vi "PH_PILS.enable extExp.vi"(0 "i ref in":refnum<vi>, 2 "Experiment.Experiment":T1(ring), 5 "error in":errorcluster) -> (14 "i ref out":refnum<vi>, 19 "error out":errorcluster)   [LabVIEW 2014, in "PH_PILS.lvlib"]
uses:
  PH_PILS.lvlib
  PH_Common/PH_Common.lvlib
  PH_SystemInformation/PH_SystemInformation.lvlib
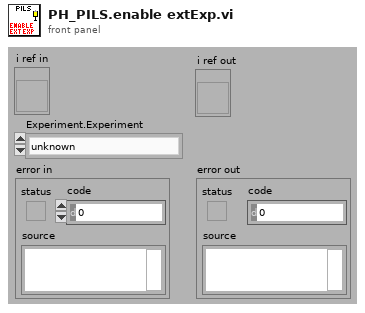
[diagram p1: front panel]
types:
  T1 = enum16{"unknown", "intern", "4 (Z6)", "3", "2", "1"}
  T2 = enum16{"Laser", "PreAmp", "MainAmp", "Exp 1", "Exp 2", "Exp 3", "Exp 4"}
  T3 = typedef "PH_PILS.lvlib/PH_PILS.i attribute.ctl" = cluster{"Boolean":cluster{"GUI Ref":refnum<vi>, "Status":i32}[], "GUI Refs Exp. Shutters":cluster{"1":refnum<vi>, "2":refnum<vi>, "3":refnum<vi>, "4":refnum<vi>}, "Tristate2Run GUI Refs":refnum<vi>[], "EO-Likes":cluster{"GUI Ref":refnum<vi>, "Status":i32}[], "Operation Mode":cluster{"Operation Mode":T4, "GUI":cluster{"Ref State":refnum<vi>, "Ref":refnum<vi>}, "Servicemode":cluster{"Tagname":string, "Status":i32}, "Labormode":cluster{"Tagname":string, "Status":i32}, "Searchmode":cluster{"Tagname":string, "Status":i32}, "Shotmode":cluster{"Tagname":string, "Status":i32}}, "Submode":cluster{"Submode":T5, "GUI":cluster{"Ref State":refnum<vi>, "Ref":refnum<vi>}, "Submode":cluster{"Tagname":string, "Status":i32}}, "Experiment":cluster{"Experiment":enum16{"unknown", "intern", "4 (Z6)", "3", "2", "1"}, "GUI":cluster{"Ref State":refnum<vi>, "Ref":refnum<vi>}, "intern":cluster{"Tagname":string, "Status":i32}, "Exp 4":cluster{"Tagname":string, "Status":i32}, "Exp 3":cluster{"Tagname":string, "Status":i32}, "Exp 2":cluster{"Tagname":string, "Status":i32}, "Exp 1":cluster{"Tagname":string, "Status":i32}}, "TristateNormal":cluster{"GUI Ref":refnum<vi>, "Status":i32}[], "Door Tags":cluster{"GUI Ref":refnum<vi>, "Status":i32}[], "GUIlessTags":cluster{"Name":string, "Status":i32}[], "Beamline GUI Refs":refnum<vi>[], "Special Boolean":cluster{"GUI Ref":refnum<vi>, "Status":i32}[], "Laserpower":cluster{"GUI Ref":refnum<vi>, "Status":i32}[], "Shutter":cluster{"GUI Ref":refnum<vi>, "Status":i32}[], "Tristate EO Like":cluster{"GUI Ref":refnum<vi>, "Status":i32}[], "PP":cluster{"GUI Ref":refnum<vi>, "Status":i32, "Head Ref":refnum<vi>, "Slider Ref":refnum<vi>}[], "Switch Knobs":cluster{"GUI Ref":refnum<vi>, "Status":i32}[], "Latch Knob GUI Refs":refnum<vi>[], "FailureCounter":i32, "Enabled Status":cluster{"Laser":i32, "PreAmp":i32, "MainAmp":i32}, "Mercury":refnum<vi>, "Instance Rods":string, "Logfile":path, "Beckhoff-Instance Internal":string, "Beckhoff-Instance External":string, "Enabling Rights":cluster{"Name":string, "Password":string, "PA?":bool, "MA?":bool, "Exp?":bool}[]}
  T4 = typedef "PH_PILS.lvlib/PH_PILS.Operation Mode.ctl" = enum16{"unknown", "Service", "Labor", "Search", "Shot"}
  T5 = typedef "PH_PILS.lvlib/PH_PILS.Submode.ctl" = enum16{"unknown", "HV-Normal", "HV-Test"}
  T6 = typedef "PH_SystemInformation.lvlib/PH_SystemInformationEnabling State.ctl" = i32
  T7 = typedef "PH_SystemInformation.lvlib/PH_SystemInformation.i attribute.ctl" = cluster{"Laser Enabling":cluster{"GUI Ref":refnum<vi>, "Enabling State":T6}, "PreAmp Enabling":cluster{"GUI Ref":refnum<vi>, "Enabling State":T6}, "MainAmp Enabling":cluster{"GUI Ref":refnum<vi>, "Enabling State":T6}, "Emergency Off":cluster{"GUI Ref":refnum<vi>, "State":enum16{"no info", "off/false", "Alarm"}}, "Enabling Exp. 1":cluster{"GUI Ref":refnum<vi>, "Enabling State":T6}, "Enabling Exp. 2":cluster{"GUI Ref":refnum<vi>, "Enabling State":T6}, "Enabling Exp. 3":cluster{"GUI Ref":refnum<vi>, "Enabling State":T6}, "Enabling Exp. 4":cluster{"GUI Ref":refnum<vi>, "Enabling State":T6}, "Timing Mode":cluster{"GUI Ref":refnum<vi>, "PHELIX_Timing_Mode":enum32{"10 Hz", "0.5 Hz", "Shot"}}}
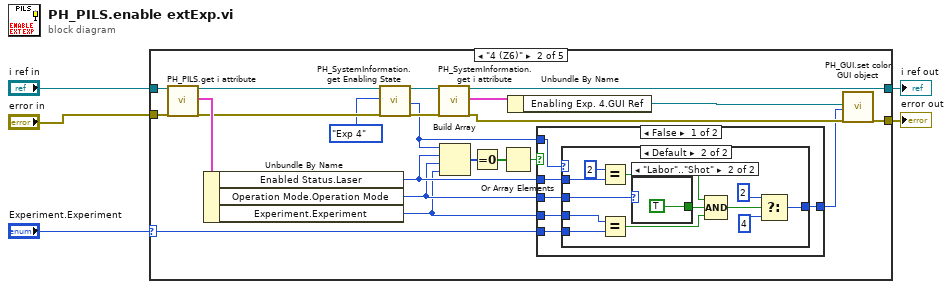
[diagram p0: block diagram]
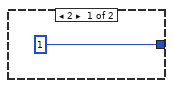
[diagram p3: hidden frame]
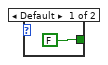
[diagram p4: hidden frame]
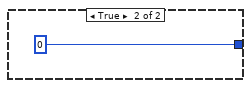
[diagram p5: hidden frame]
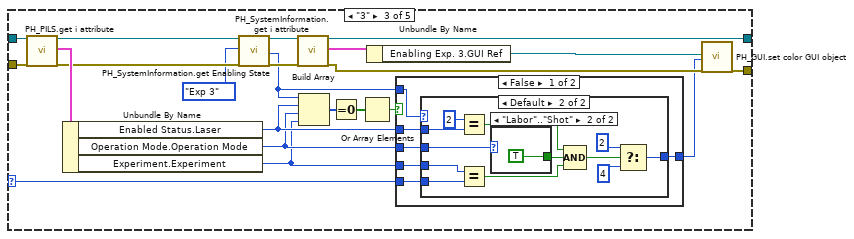
[diagram p6: hidden frame]
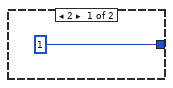
[diagram p7: hidden frame]
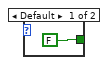
[diagram p8: hidden frame]
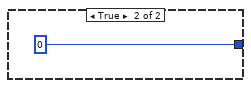
[diagram p9: hidden frame]
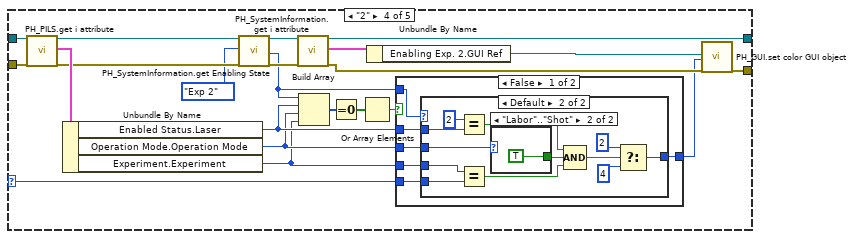
[diagram p10: hidden frame]
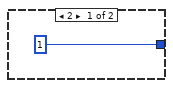
[diagram p11: hidden frame]
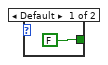
[diagram p12: hidden frame]
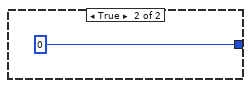
[diagram p13: hidden frame]
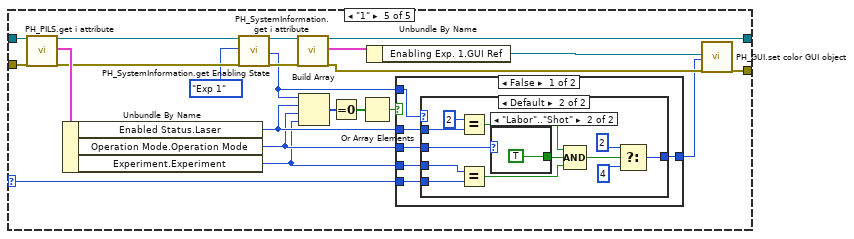
[diagram p14: hidden frame]
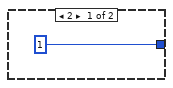
[diagram p15: hidden frame]
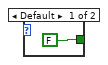
[diagram p16: hidden frame]
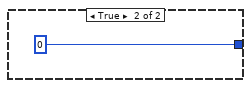
[diagram p17: hidden frame]
diagram:
  n1 = case shown="\"4 (Z6)\"" "Experiment.Experiment" {
    selector: "Experiment.Experiment" -> [_ w9 w53 w97 w141]
    tunnel: "i ref in" -> [w7 w29 w73 w117 w161]
    tunnel: "error in" -> [w6 w28 w72 w116 w160]
    tunnel: [w6 w25 w69 w113 w157] -> w3
    tunnel: [w7 w12 w56 w100 w144] -> w2
    frame Default {
    }
    frame "4 (Z6)" {
      n2 = call "PH_PILS.get i attribute.vi"("i ref in"=w29, "error in (no error)"=w28) -> ("i ref out"=w26:refnum<vi>, "i attribute"=w27:T3, "error out"=w16:errorcluster)  [unwired: 15 in]
      n3 = Unbundle By Name(w27) -> ("Enabled Status.Laser"=w23:i32, "Operation Mode.Operation Mode"=w22:T4, "Experiment.Experiment"=w21:T1)
      n4 = call "PH_SystemInformation.get Enabling State.vi"("i ref in"=w26, "Wanted State"=T2."Exp 4", "error in (no error)"=w16) -> ("i ref out"=w13:refnum<vi>, "Enabling State"=w14:T6, "error out"=w15:errorcluster)  [unwired: 14 in]
      n5 = call "PH_SystemInformation.get i attribute.vi"("i ref in"=w13, "error in (no error)"=w15) -> ("i ref out"=w12:refnum<vi>, "i attribute"=w11:T7, "error out"=w24:errorcluster)  [unwired: 15 in]
      n6 = Build Array(w14, w23, w22, w21) -> (w20:T6[])
      n7 = Equal To 0?(x=w20) -> (x = 0?=w19:bool[])
      n8 = Or Array Elements(Boolean array=w19) -> (logical OR=w18:bool)
      n9 = Unbundle By Name(w11) -> ("Enabling Exp. 4.GUI Ref"=w10:refnum<vi>)
      n10 = case shown="False" w18 {
        tunnel: [w34 0 ("State")] -> w17
        tunnel: w14 -> [w35 _]
        tunnel: w23 -> [w33 _]
        tunnel: w22 -> [w32 _]
        tunnel: w21 -> [w31 _]
        tunnel: w9 -> [w30 _]
        frame False {
          n11 = case shown="Default" w35 {
            tunnel: [1 ("State") w38] -> w34
            tunnel: w33 -> [_ w48]
            tunnel: w32 -> [_ w46]
            tunnel: w31 -> [_ w45]
            tunnel: w30 -> [_ w44]
            frame 2 {
            }
            frame Default {
              n12 = Equal?(x=2, y=w48) -> (x = y?=w43:bool)
              n13 = Equal?(x=w45, y=w44) -> (x = y?=w41:bool)
              n14 = case shown="\"Labor\"..\"Shot\"" w46 {
                tunnel: [FALSE TRUE] -> w42
                frame Default {
                }
                frame "Labor".."Shot" {
                }
              }
              n15 = Compound Arithmetic op=AND(w43, w42, w41) -> (w40:bool)
              n16 = Select(t=2 ("State"), s=w40, f=4 ("State")) -> (s? t:f=w38:i32)
            }
          }
        }
        frame True {
        }
      }
      n17 = call "PH_GUI.set color GUI object.vi"("GUI object Ref"=w10, "State"=w17, "error in (no error)"=w24) -> ("error out"=w25:errorcluster)  [unwired: 16 in]
    }
    frame "3" {
      n18 = call "PH_PILS.get i attribute.vi"("i ref in"=w73, "error in (no error)"=w72) -> ("i ref out"=w70:refnum<vi>, "i attribute"=w71:T3, "error out"=w60:errorcluster)  [unwired: 15 in]
      n19 = Unbundle By Name(w71) -> ("Enabled Status.Laser"=w67:i32, "Operation Mode.Operation Mode"=w66:T4, "Experiment.Experiment"=w65:T1)
      n20 = call "PH_SystemInformation.get Enabling State.vi"("i ref in"=w70, "Wanted State"=T2."Exp 3", "error in (no error)"=w60) -> ("i ref out"=w57:refnum<vi>, "Enabling State"=w58:T6, "error out"=w59:errorcluster)  [unwired: 14 in]
      n21 = call "PH_SystemInformation.get i attribute.vi"("i ref in"=w57, "error in (no error)"=w59) -> ("i ref out"=w56:refnum<vi>, "i attribute"=w55:T7, "error out"=w68:errorcluster)  [unwired: 15 in]
      n22 = Build Array(w58, w67, w66, w65) -> (w64:T6[])
      n23 = Equal To 0?(x=w64) -> (x = 0?=w63:bool[])
      n24 = Or Array Elements(Boolean array=w63) -> (logical OR=w62:bool)
      n25 = Unbundle By Name(w55) -> ("Enabling Exp. 3.GUI Ref"=w54:refnum<vi>)
      n26 = case shown="False" w62 {
        tunnel: [w78 0 ("State")] -> w61
        tunnel: w58 -> [w79 _]
        tunnel: w67 -> [w77 _]
        tunnel: w66 -> [w76 _]
        tunnel: w65 -> [w75 _]
        tunnel: w53 -> [w74 _]
        frame False {
          n27 = case shown="Default" w79 {
            tunnel: [1 ("State") w82] -> w78
            tunnel: w77 -> [_ w92]
            tunnel: w76 -> [_ w90]
            tunnel: w75 -> [_ w89]
            tunnel: w74 -> [_ w88]
            frame 2 {
            }
            frame Default {
              n28 = Equal?(x=2, y=w92) -> (x = y?=w87:bool)
              n29 = Equal?(x=w89, y=w88) -> (x = y?=w85:bool)
              n30 = case shown="\"Labor\"..\"Shot\"" w90 {
                tunnel: [FALSE TRUE] -> w86
                frame Default {
                }
                frame "Labor".."Shot" {
                }
              }
              n31 = Compound Arithmetic op=AND(w87, w86, w85) -> (w84:bool)
              n32 = Select(t=2 ("State"), s=w84, f=4 ("State")) -> (s? t:f=w82:i32)
            }
          }
        }
        frame True {
        }
      }
      n33 = call "PH_GUI.set color GUI object.vi"("GUI object Ref"=w54, "State"=w61, "error in (no error)"=w68) -> ("error out"=w69:errorcluster)  [unwired: 16 in]
    }
    frame "2" {
      n34 = call "PH_PILS.get i attribute.vi"("i ref in"=w117, "error in (no error)"=w116) -> ("i ref out"=w114:refnum<vi>, "i attribute"=w115:T3, "error out"=w104:errorcluster)  [unwired: 15 in]
      n35 = Unbundle By Name(w115) -> ("Enabled Status.Laser"=w111:i32, "Operation Mode.Operation Mode"=w110:T4, "Experiment.Experiment"=w109:T1)
      n36 = call "PH_SystemInformation.get Enabling State.vi"("i ref in"=w114, "Wanted State"=T2."Exp 2", "error in (no error)"=w104) -> ("i ref out"=w101:refnum<vi>, "Enabling State"=w102:T6, "error out"=w103:errorcluster)  [unwired: 14 in]
      n37 = call "PH_SystemInformation.get i attribute.vi"("i ref in"=w101, "error in (no error)"=w103) -> ("i ref out"=w100:refnum<vi>, "i attribute"=w99:T7, "error out"=w112:errorcluster)  [unwired: 15 in]
      n38 = Build Array(w102, w111, w110, w109) -> (w108:T6[])
      n39 = Equal To 0?(x=w108) -> (x = 0?=w107:bool[])
      n40 = Or Array Elements(Boolean array=w107) -> (logical OR=w106:bool)
      n41 = Unbundle By Name(w99) -> ("Enabling Exp. 2.GUI Ref"=w98:refnum<vi>)
      n42 = case shown="False" w106 {
        tunnel: [w122 0 ("State")] -> w105
        tunnel: w102 -> [w123 _]
        tunnel: w111 -> [w121 _]
        tunnel: w110 -> [w120 _]
        tunnel: w109 -> [w119 _]
        tunnel: w97 -> [w118 _]
        frame False {
          n43 = case shown="Default" w123 {
            tunnel: [1 ("State") w126] -> w122
            tunnel: w121 -> [_ w136]
            tunnel: w120 -> [_ w134]
            tunnel: w119 -> [_ w133]
            tunnel: w118 -> [_ w132]
            frame 2 {
            }
            frame Default {
              n44 = Equal?(x=2, y=w136) -> (x = y?=w131:bool)
              n45 = Equal?(x=w133, y=w132) -> (x = y?=w129:bool)
              n46 = case shown="\"Labor\"..\"Shot\"" w134 {
                tunnel: [FALSE TRUE] -> w130
                frame Default {
                }
                frame "Labor".."Shot" {
                }
              }
              n47 = Compound Arithmetic op=AND(w131, w130, w129) -> (w128:bool)
              n48 = Select(t=2 ("State"), s=w128, f=4 ("State")) -> (s? t:f=w126:i32)
            }
          }
        }
        frame True {
        }
      }
      n49 = call "PH_GUI.set color GUI object.vi"("GUI object Ref"=w98, "State"=w105, "error in (no error)"=w112) -> ("error out"=w113:errorcluster)  [unwired: 16 in]
    }
    frame "1" {
      n50 = call "PH_PILS.get i attribute.vi"("i ref in"=w161, "error in (no error)"=w160) -> ("i ref out"=w158:refnum<vi>, "i attribute"=w159:T3, "error out"=w148:errorcluster)  [unwired: 15 in]
      n51 = Unbundle By Name(w159) -> ("Enabled Status.Laser"=w155:i32, "Operation Mode.Operation Mode"=w154:T4, "Experiment.Experiment"=w153:T1)
      n52 = call "PH_SystemInformation.get Enabling State.vi"("i ref in"=w158, "Wanted State"=T2."Exp 1", "error in (no error)"=w148) -> ("i ref out"=w145:refnum<vi>, "Enabling State"=w146:T6, "error out"=w147:errorcluster)  [unwired: 14 in]
      n53 = call "PH_SystemInformation.get i attribute.vi"("i ref in"=w145, "error in (no error)"=w147) -> ("i ref out"=w144:refnum<vi>, "i attribute"=w143:T7, "error out"=w156:errorcluster)  [unwired: 15 in]
      n54 = Build Array(w146, w155, w154, w153) -> (w152:T6[])
      n55 = Equal To 0?(x=w152) -> (x = 0?=w151:bool[])
      n56 = Or Array Elements(Boolean array=w151) -> (logical OR=w150:bool)
      n57 = Unbundle By Name(w143) -> ("Enabling Exp. 1.GUI Ref"=w142:refnum<vi>)
      n58 = case shown="False" w150 {
        tunnel: [w166 0 ("State")] -> w149
        tunnel: w146 -> [w167 _]
        tunnel: w155 -> [w165 _]
        tunnel: w154 -> [w164 _]
        tunnel: w153 -> [w163 _]
        tunnel: w141 -> [w162 _]
        frame False {
          n59 = case shown="Default" w167 {
            tunnel: [1 ("State") w170] -> w166
            tunnel: w165 -> [_ w180]
            tunnel: w164 -> [_ w178]
            tunnel: w163 -> [_ w177]
            tunnel: w162 -> [_ w176]
            frame 2 {
            }
            frame Default {
              n60 = Equal?(x=2, y=w180) -> (x = y?=w175:bool)
              n61 = Equal?(x=w177, y=w176) -> (x = y?=w173:bool)
              n62 = case shown="\"Labor\"..\"Shot\"" w178 {
                tunnel: [FALSE TRUE] -> w174
                frame Default {
                }
                frame "Labor".."Shot" {
                }
              }
              n63 = Compound Arithmetic op=AND(w175, w174, w173) -> (w172:bool)
              n64 = Select(t=2 ("State"), s=w172, f=4 ("State")) -> (s? t:f=w170:i32)
            }
          }
        }
        frame True {
        }
      }
      n65 = call "PH_GUI.set color GUI object.vi"("GUI object Ref"=w142, "State"=w149, "error in (no error)"=w156) -> ("error out"=w157:errorcluster)  [unwired: 16 in]
    }
  }
  "i ref out" <- w2
  "error out" <- w3
